vi "USBFVB.vi"() -> ()   [LabVIEW 2015]
panel:
  out "Set Gate Mode":u32
  out "Shut Down":u32
  out "Detector Y Pixels":i32
  out "Get Detector":u32
  out "Get Status":u32
  out "Set Exposure Time":u32
  out "Set Trigger Mode":u32
  out "Set Readout Mode":u32
  out "Set Acquisition Mode":u32
  out "Check Timings":u32
  out "Detector X Pixels":i32
  out "Status":u32
  out "Graphical Results":i32[](graph)
  out "Start Acquisition":u32
  out "Get Acquired Data":u32
  out "Calculated Exposure Value":sgl format="%.5f"
  in  "Exposure Time (secs)":sgl format="%.2f"
  out "Initialize":u32
  in  "Trigger":u32(ring) items=["Internal", "External"]
  # "Status"
  # "Return values"
  # "USB iStar FVB32at.VI"
  # "Acquisition Mode: Single Scan\nReadout Mode: Full Vertical Binning"
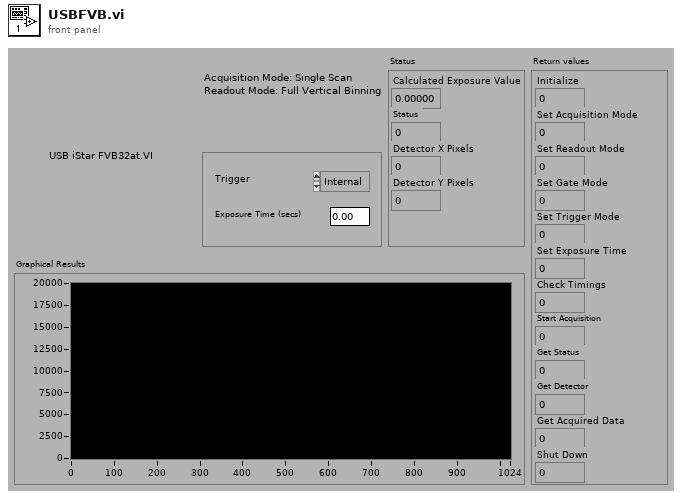
[diagram p1: front panel]
types:
  T1 = typedef "Error Code Enum typedef.ctl" = enum32{"N/A (0)", "DRV_ERROR_CODES", "DRV_SUCCESS", "DRV_VXDNOTINSTALLED", "DRV_ERROR_SCAN", "DRV_ERROR_CHECK_SUM", "DRV_ERROR_FILELOAD", "DRV_UNKNOWN_FUNC", "DRV_ERROR_VXD_INIT", "DRV_ERROR_ADDRESS", "DRV_ERROR_PAGELOCK", "DRV_ERROR_PAGEUNLOCK", "DRV_ERROR_BOARDTEST", "DRV_ERROR_ACK", "DRV_ERROR_UP_FIFO", "DRV_ERROR_PATTERN", "N/A (16)", "DRV_ACQUISITION_ERRORS", "DRV_ACQ_BUFFER", "DRV_ACQ_DOWNFIFO_FULL", "DRV_PROC_UNKONWN_INSTRUCTION", "DRV_ILLEGAL_OP_CODE", "DRV_KINETIC_TIME_NOT_MET", "DRV_ACCUM_TIME_NOT_MET", "DRV_NO_NEW_DATA", "N/A (25)", "DRV_SPOOLERROR", "N/A (27)", "N/A (28)", "N/A (29)", "N/A (30)", "N/A (31)", "N/A (32)", "DRV_TEMPERATURE_CODES", "DRV_TEMPERATURE_OFF", "DRV_TEMPERATURE_NOT_STABILIZED", "DRV_TEMPERATURE_STABILIZED", "DRV_TEMPERATURE_NOT_REACHED", "DRV_TEMPERATURE_OUT_RANGE", "DRV_TEMPERATURE_NOT_SUPPORTED", "DRV_TEMPERATURE_DRIFT", "N/A (41)", "N/A (42)", "N/A (43)", "N/A (44)", "N/A (45)", "N/A (46)", "N/A (47)", "N/A (48)", "DRV_GENERAL_ERRORS", "DRV_INVALID_AUX", "DRV_COF_NOTLOADED", "DRV_FPGAPROG", "DRV_FLEXERROR", "DRV_GPIBERROR", "N/A (55)", "N/A (56)", "N/A (57)", "N/A (58)", "N/A (59)", "N/A (60)", "N/A (61)", "N/A (62)", "N/A (63)", "DRV_DATATYPE", "DRV_DRIVER_ERRORS", "DRV_P1INVALID", "DRV_P2INVALID", "DRV_P3INVALID", "DRV_P4INVALID", "DRV_INIERROR", "DRV_COFERROR", "DRV_ACQUIRING", "DRV_IDLE", "DRV_TEMPCYCLE", "DRV_NOT_INITIALIZED", "DRV_P5INVALID", "DRV_P6INVALID", "DRV_INVALID_MODE", "DRV_INVALID_FILTER", "DRV_I2CERRORS", "DRV_I2CDEVNOTFOUND", "DRV_I2CTIMEOUT", "DRV_P7INVALID", "N/A (84)", "N/A (85)", "N/A (86)", "N/A (87)", "N/A (88)", "N/A (89)", "DRV_IOCERROR", "DRV_VRMVERSIONERROR"}
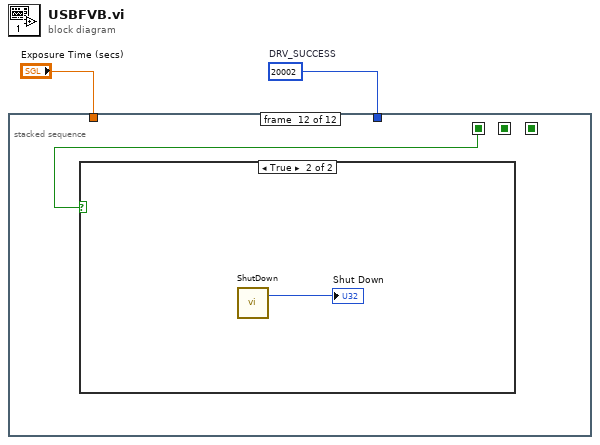
[diagram p0: block diagram]
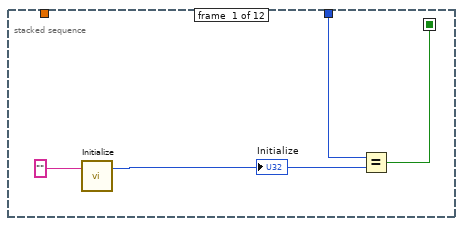
[diagram p2: hidden frame]
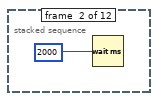
[diagram p3: hidden frame]
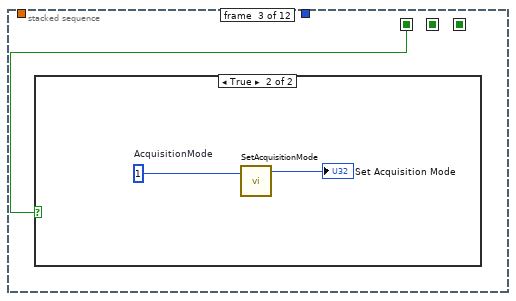
[diagram p4: hidden frame]
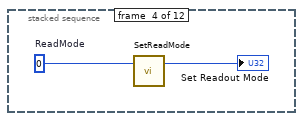
[diagram p6: hidden frame]
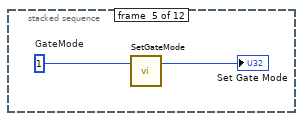
[diagram p7: hidden frame]
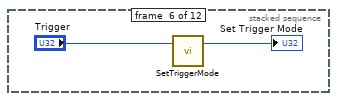
[diagram p8: hidden frame]
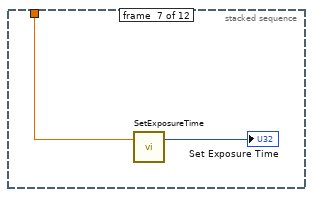
[diagram p9: hidden frame]
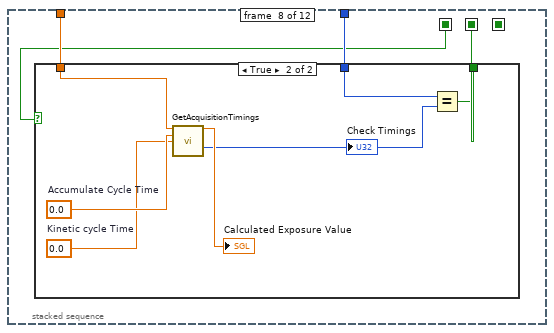
[diagram p10: hidden frame]
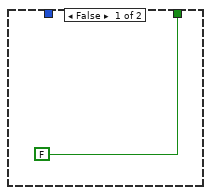
[diagram p11: hidden frame]
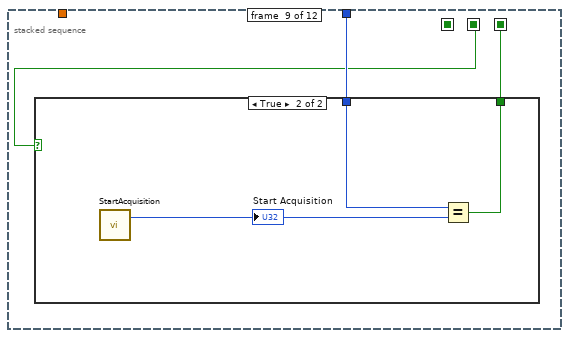
[diagram p12: hidden frame]
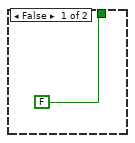
[diagram p13: hidden frame]
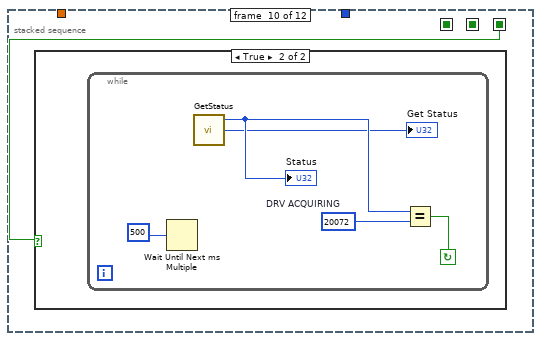
[diagram p14: hidden frame]
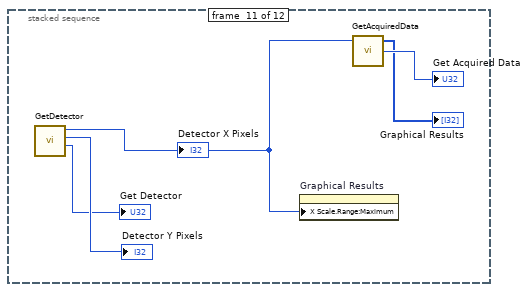
[diagram p16: hidden frame]
diagram:
  w1 = 20002  # DRV_SUCCESS
  n1 = stacked-sequence {
    seq-local: [w5 _ _ _ _ _ _ _ _ _ _ _] -> [_ _ w8 _ _ _ _ w19 _ _ _ w49]
    seq-local: [_ _ _ _ _ _ _ w20 _ _ _ _] -> [_ _ _ _ _ _ _ _ w32 _ _ _]
    seq-local: [_ _ _ _ _ _ _ _ w31 _ _ _] -> [_ _ _ _ _ _ _ _ _ w38 _ _]
    tunnel: "Exposure Time (secs)" -> [_ _ _ _ _ _ w17 w22 _ _ _ _]
    tunnel: w1 -> [w6 _ _ _ _ _ _ w21 w33 _ _ _]
    frame #0 {
      n2 = call "Initialize.vi"("directory (\"\")"="") -> ("DLL error code"=w3:u32)  [unwired: 1 in, 1 out]
      "Initialize" <- w3
      n3 = Equal?(x=w6, y=w3) -> (x = y?=w5:bool)
    }
    frame #1 {
      n4 = Wait (ms)(milliseconds to wait=u32 2000) -> ()  [unwired: 1 out]
    }
    frame #2 {
      n5 = case shown="True" w8 {
        frame False {
        }
        frame True {
          w10 = u16 1  # AcquisitionMode
          n6 = call "SetAcquisitionMode.vi"("mode"=w10) -> ("DLL error code"=→"Set Acquisition Mode":u32)  [unwired: 1 in, 1 out]
        }
      }
    }
    frame #3 {
      w11 = u16 0  # ReadMode
      n7 = call "SetReadMode.vi"("mode"=w11) -> ("DLL error code"=→"Set Readout Mode":u32)  [unwired: 1 in, 1 out]
    }
    frame #4 {
      w13 = u16 1  # GateMode
      n8 = call "SetGateMode.vi"("mode"=w13) -> ("DLL error code"=→"Set Gate Mode":u32)  [unwired: 1 in, 1 out]
    }
    frame #5 {
      n9 = call "SetTriggerMode.vi"("mode"="Trigger") -> ("DLL error code"=→"Set Trigger Mode":u32)  [unwired: 1 in, 1 out]
    }
    frame #6 {
      n10 = call "SetExposureTime.vi"("time"=w17) -> ("DLL error code"=→"Set Exposure Time":u32)  [unwired: 1 in, 1 out]
    }
    frame #7 {
      n11 = case shown="True" w19 {
        tunnel: w22 -> [_ w28]
        tunnel: w21 -> [_ w29]
        tunnel: [FALSE w30] -> w20
        frame False {
        }
        frame True {
          w27 = sgl 0.0  # Accumulate Cycle Time
          w26 = sgl 0.0  # Kinetic cycle Time
          n12 = call "GetAcquisitionTimings.vi"("exposure input"=w28, "accumulate input"=w27, "kinetic input"=w26) -> ("exposure"=→"Calculated Exposure Value":sgl, "DLL error code"=w24:u32)  [unwired: 8 in, 3 out]
          "Check Timings" <- w24
          n13 = Equal?(x=w29, y=w24) -> (x = y?=w30:bool)
        }
      }
    }
    frame #8 {
      n14 = case shown="True" w32 {
        tunnel: [FALSE w37] -> w31
        tunnel: w33 -> [_ w36]
        frame False {
        }
        frame True {
          n15 = call "StartAcquisition.vi"() -> ("DLL error code"=w35:u32)  [unwired: 2 in, 1 out]
          "Start Acquisition" <- w35
          n16 = Equal?(x=w36, y=w35) -> (x = y?=w37:bool)
        }
      }
    }
    frame #9 {
      n17 = case shown="True" w38 {
        frame False {
        }
        frame True {
          n18 = while {
            stop <- w42 continue-if-true
            w41 = u16 20072  # DRV ACQUIRING
            n19 = Wait Until Next ms Multiple(millisecond multiple=u32 500) -> ()  [unwired: 1 out]
            n20 = call "GetStatus.vi"() -> ("DLL error code"=→"Get Status":u32, "status"=w40:T1)  [unwired: 3 in, 1 out]
            "Status" <- w40
            n21 = Equal?(x=w40, y=w41) -> (x = y?=w42:bool)
          }
        }
      }
    }
    frame #10 {
      n22 = call "GetDetector.vi"() -> ("DLL error code"=→"Get Detector":u32, "ypixels"=→"Detector Y Pixels":i32, "xpixels"=w45:i32)  [unwired: 4 in, 1 out]
      "Detector X Pixels" <- w45
      n23 = property on="Graphical Results" class="WFGraph (strict)"("X Scale.Range:Maximum"=w45) -> ()  [unwired: 2 in, 2 out]
      n24 = call "GetAcquiredData.vi"("size"=w45) -> ("DLL error code"=→"Get Acquired Data":u32, "array"=→"Graphical Results":i32[])  [unwired: 2 in, 1 out]
    }
    frame #11 {
      n25 = case shown="True" w49 {
        frame False {
        }
        frame True {
          n26 = call "ShutDown.vi"() -> ("DLL error code"=→"Shut Down":u32)  [unwired: 2 in, 1 out]
        }
      }
    }
  }
